vi "LoadRobotID.vi"(1 "Robot ID File":path, 2 "DefaultRobotID":T1, 3 "OverrideFileValue":bool) -> (0 "RobotID":T1)   [LabVIEW 2019]
uses:
  TypeDefs/RobotID.ctl
  <vilib>/Utility/Data Type/NI_Data Type.lvlib
  <vilib>/Utility/file.llb/Read Delimited Spreadsheet (string).vi
  f55d2e64-4a24-448d-b373-45147090c9b5.vi
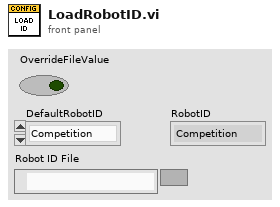
[diagram p1: front panel]
types:
  T1 = typedef "RobotID.ctl" = enum16{"Competition", "Practice"}
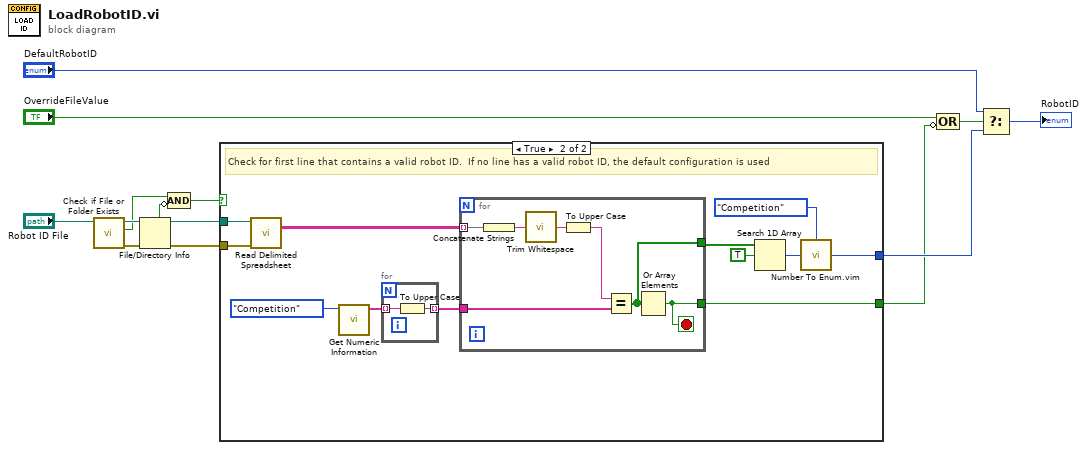
[diagram p0: block diagram]
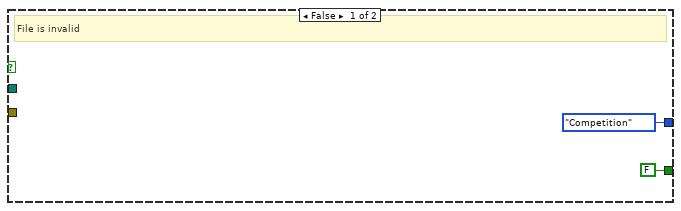
[diagram p2: hidden frame]
diagram:
  n1 = call <vilib>:"Check if File or Folder Exists.vi"("path"="Robot ID File") -> ("error out"=w8:errorcluster, "file or folder exists?"=w7:bool, "dup path"=w9:path)  [unwired: 8 in]
  n2 = File/Directory Info(path=w9, error in=w8) -> (path out=w5:path, directory=w6:bool, error out=w3:errorcluster)  [unwired: 4 out]
  n3 = Compound Arithmetic op=AND(w7, invert w6) -> (w4:bool)
  n4 = case shown="True" w4 {
    tunnel: w5 -> [_ w28]
    tunnel: w3 -> [_ w27]
    tunnel: [RobotID."Competition" ("DefaultRobotID") w19] -> w2
    tunnel: [FALSE w23] -> w1
    frame False {
      # "File is invalid"
    }
    frame True {
      # "Check for first line that contains a valid robot ID.  If no line has a valid robot ID, the default configuration is used"
      n5 = call-poly <vilib>:"Read Delimited Spreadsheet.vi"("file path (dialog if empty)"=w28, "error in (no error)"=w27) -> ("all rows"=w26:string[][])  [unwired: 8 in, 5 out]
      n6 = call <vilib>:"Get Numeric Information.vi"("variant"=RobotID."Competition" ("Robot ID")) -> ("enum names"=w25:string[])  [unwired: 7 in, 3 out]
      n7 = for {
        tunnel: w25 -> [w30] mode=indexing
        tunnel: [w29] -> w24 mode=indexing
        n8 = To Upper Case(1:w30) -> (0:w29:string)
      }
      n9 = for {
        tunnel: w26 -> [w37] mode=indexing
        tunnel: w24 -> [w34]
        tunnel: [w32] -> w23
        tunnel: [w31] -> w22
        stop <- w32 stop-if-true
        n10 = Concatenate Strings(w37) -> (w36:string)
        n11 = call <vilib>:"Trim Whitespace.vi"("string"=w36) -> ("trimmed string"=w35:string)  [unwired: 1 in]
        n12 = To Upper Case(1:w35) -> (0:w33:string)
        n13 = Equal?(x=w33, y=w34) -> (x = y?=w31:bool[])
        n14 = Or Array Elements(Boolean array=w31) -> (logical OR=w32:bool)
      }
      n15 = Search 1D Array(1D array=w22, element=TRUE) -> (index of element=w20:i32)  [unwired: 1 in]
      n16 = call "Number To Enum.vim"("number"=w20, "enum type"=RobotID."Competition" ("Robot ID")) -> ("number as enum"=w19:T1)
    }
  }
  n17 = Compound Arithmetic op=OR("OverrideFileValue", invert w1) -> (w11:bool)
  n18 = Select(t="DefaultRobotID", s=w11, f=w2) -> (s? t:f=→"RobotID":T1)
